vi "Channel_FromXML.vi"(8 "error in (no error)":errorcluster, 11 "XML String":string) -> (0 "error out":errorcluster, 3 "Channel out":refnum<class "Channel.lvclass">)   [LabVIEW 2023, in "Channel.lvclass"]
doc: "Define our channel class based on a given XML Configuration."
uses:
  Channel.lvclass
  ChannelAsCluster.ctl
  <vilib>/NI VeriStand/Custom Device API/Data Reference.ctl
  Meta Data.ctl
  <vilib>/NI VeriStand/Custom Device API/Custom Device API.lvlib
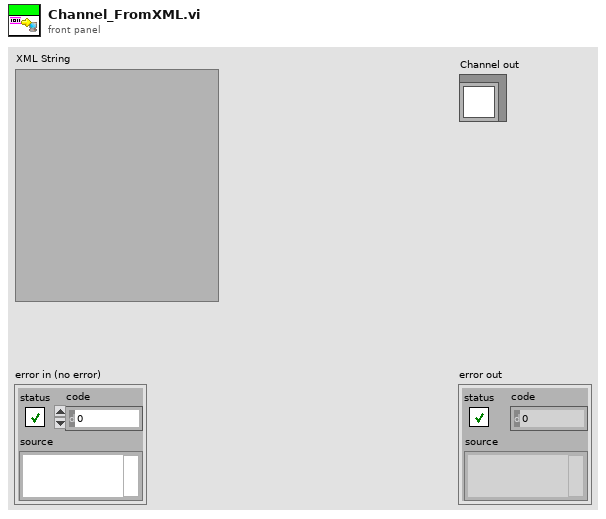
[diagram p1: front panel]
types:
  T1 = typedef "ChannelAsCluster.ctl" = cluster{"Name":string, "Data Reference":T2, "Wfm?":bool, "Decimation":i32, "Current Value":dbl, "Meta Data":T3[], "WfmPath":string}
  T2 = typedef "Custom Device API.lvlib/Data Reference.ctl" = i32
  T3 = typedef "Meta Data.ctl" = cluster{"Key":string, "Value":string}
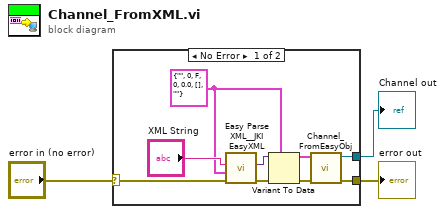
[diagram p0: block diagram]
diagram:
  n1 = case shown="No Error" "error in (no error)" {
    selector: "error in (no error)" -> [w11 w13]
    tunnel: [w4 w13] -> w2
    tunnel: [w6 _] -> w1
    frame No Error {
      w8 = T1 {"Name"="", "Data Reference"=0, "Wfm?"=FALSE, "Decimation"=0, "Current Value"=0.0, "Meta Data"=[], "WfmPath"=""} ("output cluster")
      n2 = call <vilib>:"Easy Parse XML__JKI EasyXML.vi"("error in (no error)"=w11, "LabVIEW Data (Type)"=w8, "XML String"="XML String") -> ("error out"=w9:errorcluster, "LabVIEW Data"=w10:variant)  [unwired: 7 in]
      n3 = Variant To Data(error in=w9, type=w8, Variant=w10) -> (data=w7:T1, error out=w5:errorcluster)
      n4 = call "Channel_FromEasyObj.vi"("error in (no error)"=w5, "output cluster"=w7) -> ("error out"=w4:errorcluster, "Channel out"=w6:refnum<class "Channel.lvclass">)  [unwired: 8 in]
    }
    frame Error {
    }
  }
  "error out" <- w2
  "Channel out" <- w1
